vi "Macro Command Demo.vi"() -> ()   [LabVIEW 2013]
uses:
  MacroCommand_class/MacroCommand.lvclass
  SpindleOffCommand_class/SpindleOffCommand.lvclass
  SpindleOnCommand_class/SpindleOnCommand.lvclass
  Spindle_class/Spindle.lvclass
  <vilib>/addons/_AddQ/G#Object/G#Object.lvclass
panel:
  in  "Off Comand":bool
  in  "停止":bool
  in  "On Command":bool
  out "# of objects killed 2":i32
  out "Output":string
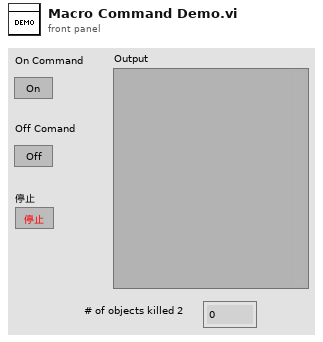
[diagram p1: front panel]
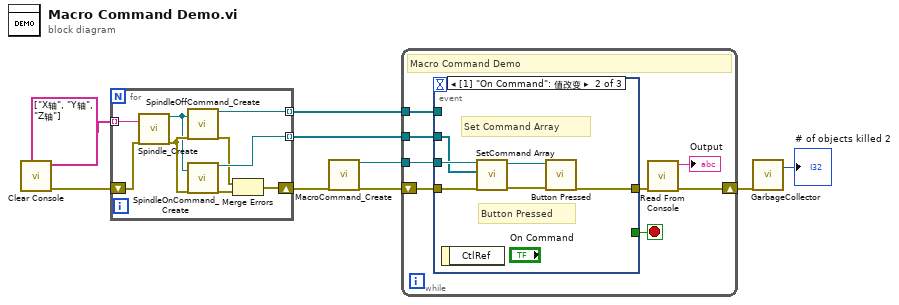
[diagram p0: block diagram]
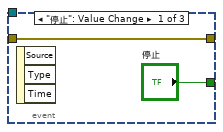
[diagram p2: hidden frame]
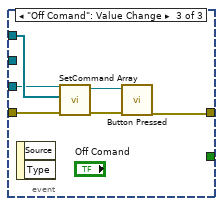
[diagram p3: hidden frame]
diagram:
  n1 = call "Clear Console.vi"() -> ("error out"=w6:errorcluster)  [unwired: 11 in]
  n2 = for {
    tunnel: string[] ["X轴", "Y轴", "Z轴"] -> [w18] mode=indexing
    tunnel: [w14] -> w3 mode=indexing
    tunnel: [w13] -> w2 mode=indexing
    shift-right: [w10] -> w5
    shift-left: w6 -> [w15]
    n3 = call "Spindle_Create.vi"("Name"=w18, "error in (no error)"=w15) -> ("reference out"=w16:refnum<class "Spindle.lvclass">, "error out"=w17:errorcluster)  [unwired: 16 in]
    n4 = call "SpindleOffCommand_Create.vi"("Spindle.lvclass"=w16, "error in (no error)"=w17) -> ("reference out"=w14:refnum<class "SpindleOffCommand.lvclass">, "error out"=w12:errorcluster)  [unwired: 16 in]
    n5 = call "SpindleOnCommand_Create.vi"("Spindle.lvclass"=w16, "error in (no error)"=w17) -> ("reference out"=w13:refnum<class "SpindleOnCommand.lvclass">, "error out"=w11:errorcluster)  [unwired: 16 in]
    n6 = Merge Errors(w12, w11) -> (w10:errorcluster)
  }
  n7 = call "MacroCommand_Create.vi"("error in (no error)"=w5) -> ("reference out"=w1:refnum<class "MacroCommand.lvclass">, "error out"=w4:errorcluster)  [unwired: 17 in]
  n8 = while {
    shift-right: [w23] -> w8
    shift-left: w4 -> [w25]
    tunnel: w3 -> [w21]
    tunnel: w2 -> [w19]
    tunnel: w1 -> [w20]
    stop <- w26 stop-if-true
    # "Macro Command Demo"
    n9 = event shown="[1] \"On Command\": 值改变" {
      selector: _ -> [_ _ _]
      dyn-events: _ -> [_ _ _]
      timeout: _ -> [_ _ _]
      tunnel: ["停止" _ _] -> w26
      tunnel: w25 -> [w27 w34 w40]
      tunnel: [w27 w29 w35] -> w24
      tunnel: w21 -> [_ _ w39]
      tunnel: w20 -> [_ w33 w38]
      tunnel: w19 -> [_ w32 _]
      event "停止": Value Change {
        n10 = event-data() -> ()  [unwired: 1 in, 3 out]
      }
      event "On Command": Value Change {
        # "Button Pressed"
        # "Set Command Array"
        n11 = event-data() -> ()  [unwired: 1 in, 1 out]
        n12 = call "SetCommand Array.vi"("error in (no error)"=w34, "Command Array"=w32, "reference in"=w33) -> ("error out"=w31:errorcluster, "reference out"=w30:refnum<class "MacroCommand.lvclass">)  [unwired: 7 in]
        n13 = call-dynamic "Button Pressed.vi"("reference in"=w30, "error in (no error)"=w31) -> ("error out"=w29:errorcluster)  [unwired: 16 in, 1 out]
      }
      event "Off Comand": Value Change {
        n14 = event-data() -> ()  [unwired: 1 in, 2 out]
        n15 = call "SetCommand Array.vi"("error in (no error)"=w40, "Command Array"=w39, "reference in"=w38) -> ("error out"=w36:errorcluster, "reference out"=w37:refnum<class "MacroCommand.lvclass">)  [unwired: 7 in]
        n16 = call-dynamic "Button Pressed.vi"("reference in"=w37, "error in (no error)"=w36) -> ("error out"=w35:errorcluster)  [unwired: 16 in, 1 out]
      }
    }
    n17 = call "Read From Console.vi"("error in (no error)"=w24) -> ("error out"=w23:errorcluster, "Output"=→"Output":string)  [unwired: 9 in]
  }
  n18 = call <vilib>:"GarbageCollector.vi"("error in (no error)"=w8) -> ("# of objects killed"=→"# of objects killed 2":i32)  [unwired: 16 in, 2 out]
